vi "Buffer Strings.vi"(6 "Insert between Strings (\"\")":string, 9 "number of strings to buffer (15)":u8=15, 11 "new string":string) -> (3 "buffered string series":string)   [LabVIEW 2015, in "Car Wash.lvlib" / "Tools_String.lvlib"]
doc: "This VI buffers and returns a series of strings using a an internal shift register. It is commonly used to display the last N strings returned form a device, instrument, process, etc. The user can select how many strings are buffered and returned from this VI. \n\nThe Insert between Strings parameter value is inserted between each of the buffered strings."
uses:
  Tools_String.lvlib
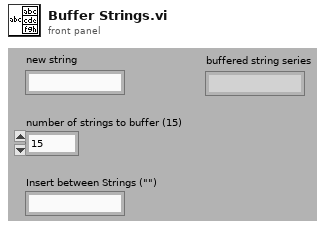
[diagram p1: front panel]
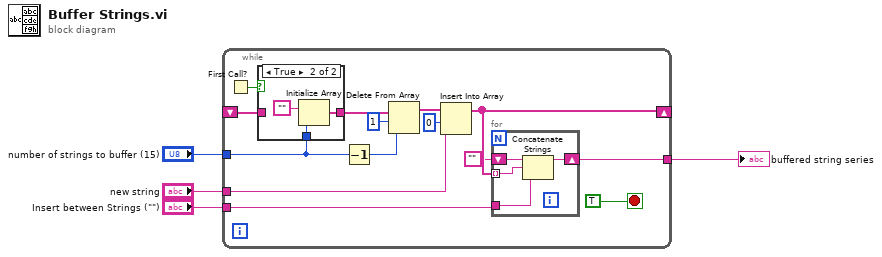
[diagram p0: block diagram]
diagram:
  n1 = while {
    shift-right: [w12] -> _
    shift-left: _ -> [w17]
    tunnel: [w8] -> w4
    tunnel: "Insert between Strings (\"\")" -> [w7]
    tunnel: "number of strings to buffer (15)" -> [w6]
    tunnel: "new string" -> [w5]
    stop <- TRUE stop-if-true
    n2 = First Call?() -> (First Call?: T/F=w18:bool)
    n3 = case shown="True" w18 {
      tunnel: [w23 w25] -> w16
      tunnel: w17 -> [w23 _]
      tunnel: w6 -> [_ w24]
      frame False {
      }
      frame True {
        n4 = Initialize Array("" ("element"), w24) -> (w25:string[])
      }
    }
    n5 = Decrement(x=w6) -> (x-1=w15:u8)
    n6 = Delete From Array(array=w16, length=1, index=w15) -> (array with subset deleted=w13:string[])  [unwired: 1 out]
    n7 = Insert Into Array(array=w13, index=0, new element=w5) -> (w12:string[])
    n8 = for {
      tunnel: w12 -> [w21] mode=indexing
      shift-right: [w20] -> w8
      shift-left: "" ("element") -> [w22]
      tunnel: w7 -> [w19]
      n9 = Concatenate Strings(w22, w21, w19) -> (w20:string)
    }
  }
  "buffered string series" <- w4
